vi "replaceNullTimes.vi"(8 "error in (no error)":errorcluster, 10 "data in":T1(array[cluster]), 11 "ScriptEventList in":refnum<class "ScriptEventList.lvclass">) -> (0 "error out":errorcluster, 2 "data out":T1(array[cluster]), 3 "ScriptEventList out":refnum<class "ScriptEventList.lvclass">)   [LabVIEW 2011, in "Tools.lvlib" / "Scripting.lvlib" / "ScriptEventList.lvclass"]
uses:
  ScriptEventList.lvclass
  DatabaseHelpers/Database Objects/Channel/Channel.lvclass
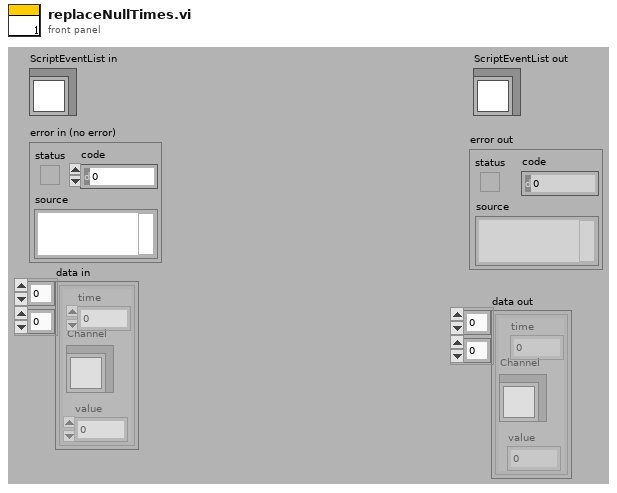
[diagram p1: front panel]
types:
  T1 = cluster{"time":dbl, "Channel":refnum<class "Channel.lvclass">, "value":dbl}[][]
  T2 = cluster{"time":dbl, "Channel":refnum<class "Channel.lvclass">, "value":dbl}
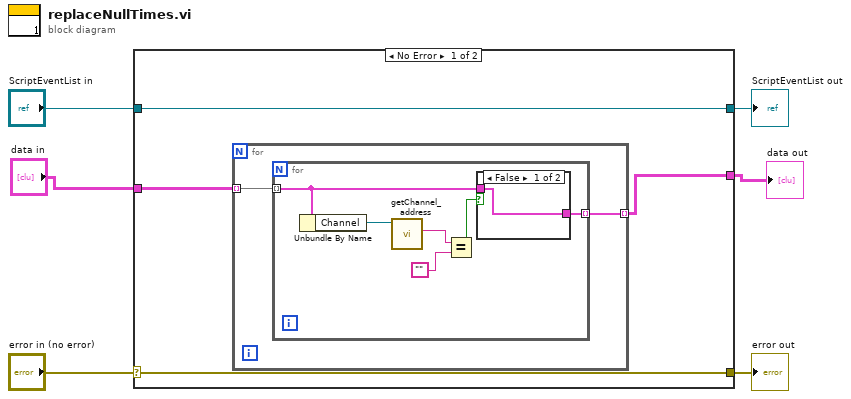
[diagram p0: block diagram]
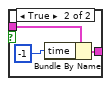
[diagram p2: hidden frame]
diagram:
  n1 = case shown="No Error" "error in (no error)" {
    selector: "error in (no error)" -> [w9 w24]
    tunnel: [w9 w24] -> w5
    tunnel: [w10 w23] -> w3
    tunnel: "ScriptEventList in" -> [w10 w23]
    tunnel: "data in" -> [w8 _]
    tunnel: [w7 _] -> w1
    frame No Error {
      n2 = for {
        tunnel: w8 -> [w12] mode=indexing
        tunnel: [w11] -> w7 mode=indexing
        n3 = for {
          tunnel: w12 -> [w15] mode=indexing
          tunnel: [w14] -> w11 mode=indexing
          n4 = Unbundle By Name(w15) -> ("Channel"=w18:refnum<class "Channel.lvclass">)
          n5 = call "getChannel_address.vi"("Channel.lvclass in"=w18) -> ("channel_address"=w16:string)  [unwired: 8 in, 2 out]
          n6 = Equal?(x=w16, y="") -> (x = y?=w13:bool)
          n7 = case shown="False" w13 {
            tunnel: w15 -> [w19 w22]
            tunnel: [w19 w20] -> w14
            frame False {
            }
            frame True {
              n8 = Bundle By Name(cluster=w22, "time"=-1) -> (w20:T2)
            }
          }
        }
      }
    }
    frame Error {
    }
  }
  "error out" <- w5
  "ScriptEventList out" <- w3
  "data out" <- w1
